vi "split_doses.vi"(0 "Volume":dbl format="%_4f") -> (1 "Doses":string[](array[string]), 2 "Coerced?":bool, 3 "OutVolume":dbl)   [LabVIEW 2010]
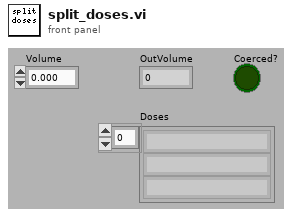
[diagram p1: front panel]
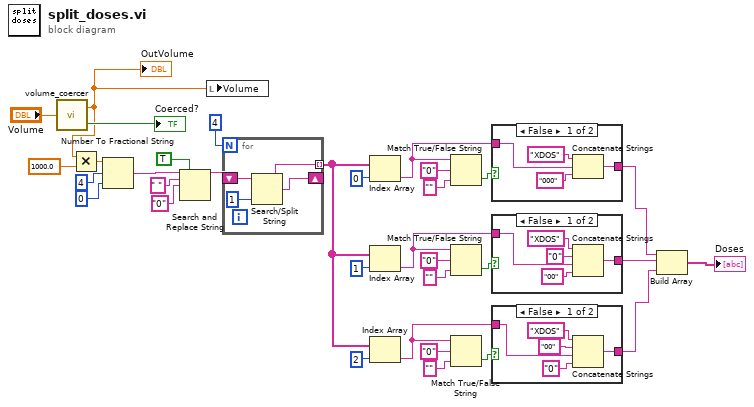
[diagram p0: block diagram]
diagram:
  n1 = call "volume_coercer.vi"("InVolume"="Volume") -> ("OutVolume"=w29:dbl, "Coerced?"=→"Coerced?":bool)
  "OutVolume" <- w29
  n2 = Multiply(x=w29, y=1000.0) -> (x*y=w3:dbl)
  n3 = Number To Fractional String(number=w3, width (-)=i16 4, precision (6)=i16 0) -> (F-format string=w6:string)  [unwired: 1 in]
  n4 = Search and Replace String(replace all?=TRUE ("replace all? (F)"), input string=w6, search string=" " ("substring (\"\")"), replace string="0" ("replace string (\"\")")) -> (result string=w10:string)  [unwired: 4 in, 3 out]
  n5 = local write "Volume"(w29) -> ()
  n6 = for {
    N: 4 ("Numeric") -> [_]
    shift-right: [w35] -> _
    shift-left: w10 -> [w37]
    tunnel: [w34] -> w27 mode=indexing
    n7 = Search/Split String(string=w37, offset (0)=1) -> (substring before match=w34:string, match + rest of string=w35:string)  [unwired: 1 in, 1 out]
  }
  n8 = Index Array(array=w27, index=0) -> (element=w16:string)
  n9 = Index Array(array=w27, index=1) -> (element=w17:string)
  n10 = Index Array(array=w27, index=2) -> (element=w26:string)
  n11 = Match True/False String(2:"" ("false string"), 3:"0" ("true string"), 4:w16) -> (0:w14:bool)  [unwired: 1 out]
  n12 = Match True/False String(2:"" ("false string"), 3:"0" ("true string"), 4:w17) -> (0:w19:bool)  [unwired: 1 out]
  n13 = Match True/False String(2:"" ("false string"), 3:"0" ("true string"), 4:w26) -> (0:w24:bool)  [unwired: 1 out]
  n14 = case shown="False" w14 {
    tunnel: w16 -> [w40 _]
    tunnel: [w38 _] -> w33
    frame False {
      n15 = Concatenate Strings("XDOS" ("string"), w40, "000" ("string")) -> (w38:string)
    }
    frame True {
    }
  }
  n16 = case shown="False" w19 {
    tunnel: w17 -> [w44 _]
    tunnel: [w42 _] -> w31
    frame False {
      n17 = Concatenate Strings("XDOS" ("string"), "0" ("string"), w44, "00" ("string")) -> (w42:string)
    }
    frame True {
    }
  }
  n18 = case shown="False" w24 {
    tunnel: w26 -> [w48 _]
    tunnel: [w47 _] -> w32
    frame False {
      n19 = Concatenate Strings("XDOS" ("string"), "00" ("string"), w48, "0" ("string")) -> (w47:string)
    }
    frame True {
    }
  }
  n20 = Build Array(w33, w31, w32) -> (→"Doses":string[])
